vi "RS-Glied.vi"(8 "reset":bool, 11 "set":bool) -> (1 "Fehler":bool)   [LabVIEW 2020, in "Erweiterte Konfig.lvlib" / "CG-Check Konfig.lvlib"]
uses:
  CG-Check Konfig.lvlib
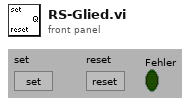
[diagram p1: front panel]
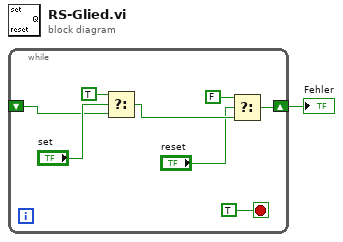
[diagram p0: block diagram]
diagram:
  n1 = while {
    shift-right: [w3] -> w1
    shift-left: _ -> [w2]
    stop <- TRUE stop-if-true
    n2 = Select(t=TRUE, s="set", f=w2) -> (s? t:f=w5:bool)
    n3 = Select(t=FALSE, s="reset", f=w5) -> (s? t:f=w3:bool)
  }
  "Fehler" <- w1
